vi "Filter Depth.vi"(6 "Wall-Threshold":i32=150, 8 "Y-Threshold":i32=150, 9 "Far object filter":i32(slide)=26869 scale=0.0..7000.0, 10 "Depth Image Pixels (U16)":u16[][](array[numeric]), 11 "Replace with?":i32=60000) -> (0 "average Z":dbl, 1 "average Y":dbl, 2 "average X":dbl, 3 "Array":i32[][](array[numeric]), 4 "New far object filter":i32, 5 "Area":i32)   [LabVIEW 2011, in "Kinect_API.lvlib"]
uses:
  Kinect_API.lvlib
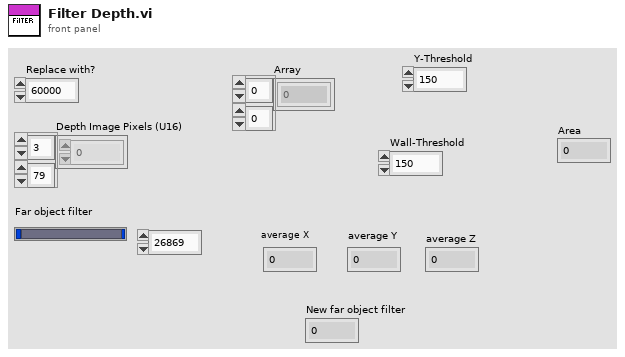
[diagram p1: front panel]
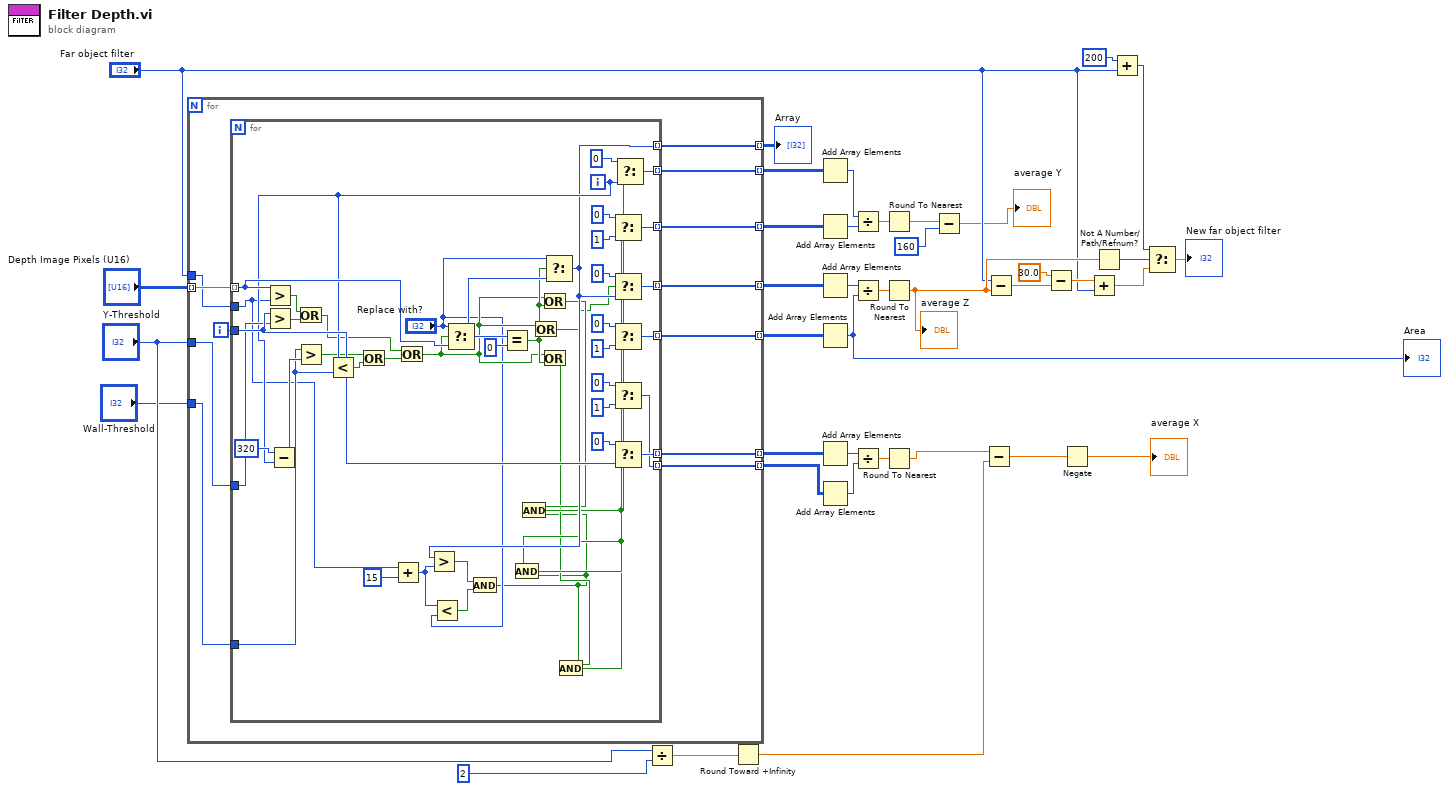
[diagram p0: block diagram]
diagram:
  n1 = for {
    tunnel: "Depth Image Pixels (U16)" -> [w50] mode=indexing
    tunnel: [w49] -> w38 mode=indexing
    tunnel: [w48] -> w36 mode=indexing
    tunnel: [w47] -> w35 mode=indexing
    tunnel: [w45] -> w30 mode=indexing
    tunnel: [w44] -> w29 mode=indexing
    tunnel: [w43] -> w26 mode=indexing
    tunnel: [w42] -> w25 mode=indexing
    tunnel: "Far object filter" -> [w41]
    tunnel: "Y-Threshold" -> [w40]
    tunnel: "Wall-Threshold" -> [w39]
    i -> [w46]
    n2 = for {
      tunnel: w50 -> [w96] mode=indexing
      tunnel: [w64] -> w49 mode=indexing
      tunnel: [w92] -> w48 mode=indexing
      tunnel: [w89] -> w47 mode=indexing
      tunnel: w46 -> [w76]
      tunnel: [w85] -> w45 mode=indexing
      tunnel: [w84] -> w44 mode=indexing
      tunnel: [w80] -> w43 mode=indexing
      tunnel: [w79] -> w42 mode=indexing
      tunnel: w41 -> [w63]
      tunnel: w40 -> [w75]
      tunnel: w39 -> [w71]
      i -> [w72]
      n3 = Greater?(x=w96, y=w63) -> (0:w77:bool)
      n4 = Greater?(x=w76, y=w75) -> (0:w78:bool)
      n5 = Subtract(x=320 ("y"), y=w72) -> (x-y=w73:i32)
      n6 = Or(x=w77, y=w78) -> (x .or. y?=w68:bool)
      n7 = Greater?(x=w71, y=w73) -> (0:w70:bool)
      n8 = Less?(x=w72, y=w71) -> (x < y?=w69:bool)
      n9 = Or(x=w70, y=w69) -> (x .or. y?=w67:bool)
      n10 = Add(x=w63, y=15) -> (x+y=w61:i32)
      n11 = Or(x=w68, y=w67) -> (x .or. y?=w65:bool)
      n12 = Less?(x=w61, y="Replace with?") -> (x < y?=w59:bool)
      n13 = Select(t="Replace with?", s=w65, f=w96) -> (s? t:f=w94:i32)
      n14 = Equal?(x=w94, y=0) -> (x = y?=w66:bool)
      n15 = Or(x=w65, y=w66) -> (x .or. y?=w54:bool)
      n16 = Or(x=w65, y=w66) -> (x .or. y?=w57:bool)
      n17 = Or(x=w65, y=w66) -> (x .or. y?=w52:bool)
      n18 = Select(t="Replace with?", s=w66, f=w94) -> (s? t:f=w64:i32)
      n19 = Greater?(x=w64, y=w61) -> (0:w58:bool)
      n20 = And(x=w58, y=w59) -> (x .and. y?=w51:bool)
      n21 = And(x=w54, y=w51) -> (x .and. y?=w55:bool)
      n22 = And(x=w57, y=w51) -> (x .and. y?=w56:bool)
      n23 = And(x=w52, y=w51) -> (x .and. y?=w53:bool)
      n24 = Select(t=0, s=w56, f=1) -> (s? t:f=w79:i32)
      n25 = Select(t=0, s=w55, f=w64) -> (s? t:f=w92:i32)
      n26 = Select(t=0, s=w55, f=1) -> (s? t:f=w89:i32)
      n27 = Select(t=0, s=w53, f=1) -> (s? t:f=w84:i32)
      n28 = Select(t=0, s=w53, f=w76) -> (s? t:f=w85:i32)
      n29 = Select(t=0, s=w56, f=w72) -> (s? t:f=w80:i32)
    }
  }
  "Array" <- w38
  n30 = Divide(x="Y-Threshold", y=2) -> (x/y=w10:dbl)
  n31 = Round Toward +Infinity(x=w10) -> (ceil(x): smallest int >= x=w7:dbl)
  n32 = Add Array Elements(numeric array=w26) -> (sum=w28:i32)
  n33 = Add Array Elements(numeric array=w25) -> (sum=w27:i32)
  n34 = Add Array Elements(numeric array=w36) -> (sum=w34:i32)
  n35 = Add Array Elements(numeric array=w35) -> (sum=w33:i32)
  "Area" <- w33
  n36 = Add Array Elements(numeric array=w30) -> (sum=w32:i32)
  n37 = Add Array Elements(numeric array=w29) -> (sum=w31:i32)
  n38 = Divide(x=w28, y=w27) -> (x/y=w12:dbl)
  n39 = Divide(x=w34, y=w33) -> (x/y=w24:dbl)
  n40 = Divide(x=w32, y=w31) -> (x/y=w23:dbl)
  n41 = Round To Nearest(number=w12) -> (nearest integer value=w11:dbl)
  n42 = Round To Nearest(number=w24) -> (nearest integer value=w19:dbl)
  "average Z" <- w19
  n43 = Round To Nearest(number=w23) -> (nearest integer value=w8:dbl)
  n44 = Subtract(x=w11, y=160) -> (x-y=→"average Y":dbl)
  n45 = Subtract(x=w8, y=w7) -> (x-y=w4:dbl)
  n46 = Subtract(x="Far object filter", y=w19) -> (x-y=w21:dbl)
  n47 = Subtract(x=30.0 ("y"), y=w21) -> (x-y=w20:dbl)
  n48 = Negate(x=w4) -> (-x=→"average X":dbl)
  n49 = Add(x=w20, y="Far object filter") -> (x+y=w16:dbl)
  n50 = Not A Number/Path/Refnum?(number/path/refnum=w19) -> (NaN/Path/Refnum?=w17:bool)
  n51 = Add(x=200, y="Far object filter") -> (x+y=w15:i32)
  n52 = Select(t=w15, s=w17, f=w16) -> (s? t:f=→"New far object filter":dbl)
